vi "create_log_file.vi"(8 "error in (no error)":errorcluster caption="错误输入（无错误）", 11 "Log 输入":refnum<class "Log.lvclass">) -> (0 "error out":errorcluster caption="错误输出", 3 "Log 输出":refnum<class "Log.lvclass">)   [LabVIEW 2018, in "Log.lvlib" / "Log.lvclass"]
uses:
  Log.lvclass
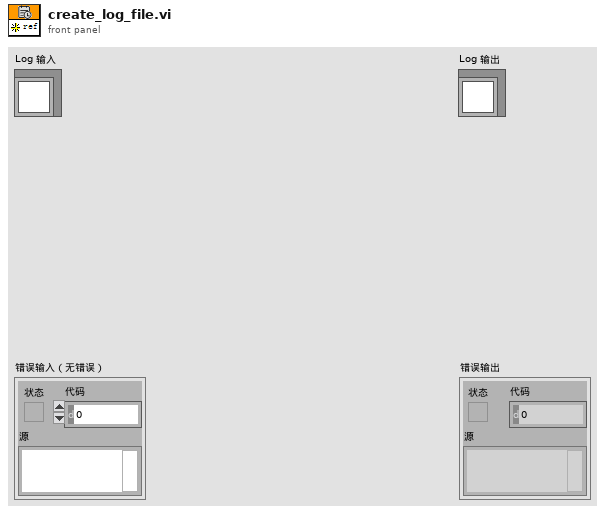
[diagram p1: front panel]
types:
  T1 = enum16{"open", "replace", "create", "open or create", "replace or create", "replace or create with confirmation"}
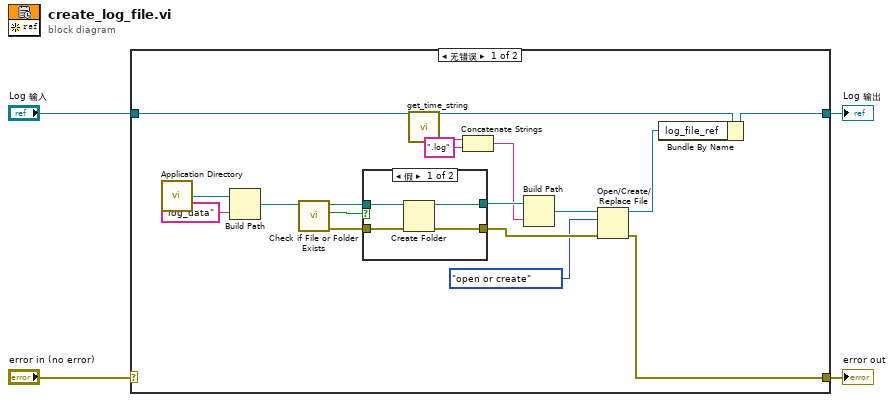
[diagram p0: block diagram]
diagram:
  n1 = case shown="无错误" "error in (no error)" {
    selector: "error in (no error)" -> [_ w29]
    tunnel: [w10 w29] -> w3
    tunnel: [w8 w28] -> w1
    tunnel: "Log 输入" -> [w21 w28]
    frame No Error {
      n2 = call <vilib>:"Application Directory.vi"() -> ("Application Directory"=w20:path)
      n3 = Build Path(base path=w20, name or relative path="log_data" ("名称或相对路径")) -> (appended path=w18:path)
      n4 = call <vilib>:"Check if File or Folder Exists.vi"("path"=w18) -> ("error out"=w15:errorcluster, "file or folder exists?"=w17:bool, "dup path"=w16:path)  [unwired: 8 in]
      n5 = case shown="假" w17 {
        tunnel: w16 -> [w25 w27]
        tunnel: w15 -> [w24 w26]
        tunnel: [w23 w27] -> w14
        tunnel: [w22 w26] -> w12
        frame False {
          n6 = Create Folder(path (use dialog)=w25, error in=w24) -> (created path=w23:path, error out=w22:errorcluster)  [unwired: 1 in, 1 out]
        }
        frame True {
        }
      }
      n7 = call "get_time_string.vi"() -> ("date/time string"=w13:string)  [unwired: 11 in]
      n8 = Concatenate Strings(w13, ".log" ("字符串")) -> (w6:string)
      n9 = Build Path(base path=w14, name or relative path=w6) -> (appended path=w11:path)
      n10 = Open/Create/Replace File(file path (use dialog)=w11, error in=w12, operation (0:open)=T1."open or create" ("操作(0:open)")) -> (refnum out=w7:refnum<file>, error out=w10:errorcluster)  [unwired: 3 in, 1 out]
      n11 = Bundle By Name(cluster=w21, "log_file_ref"=w7) -> (w8:refnum<class "Log.lvclass">)
    }
    frame Error {
    }
  }
  "error out" <- w3
  "Log 输出" <- w1
